vi "Ramp Down R1.vi"(10 "V":dbl, 11 "Refnum in":refnum<k20>) -> (3 "Refnum out":refnum<k20>)   [LabVIEW 2018]
uses:
  <vilib>/Utility/error.llb/Error Cluster From Error Code.vi
  <vilib>/rvi/errors/niLvFpgaAdjustHostInterfaceError.vi
  <vilib>/rvi/interface/nirviReadWriteControl/nirviReadWriteControl.xnode
  NiFpgaLv.dll
  <vilib>/rvi/interface/Simulation/niFpgaSimulationCallBeginRW.vi
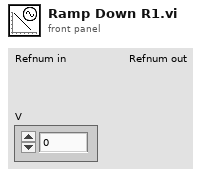
[diagram p1: front panel]
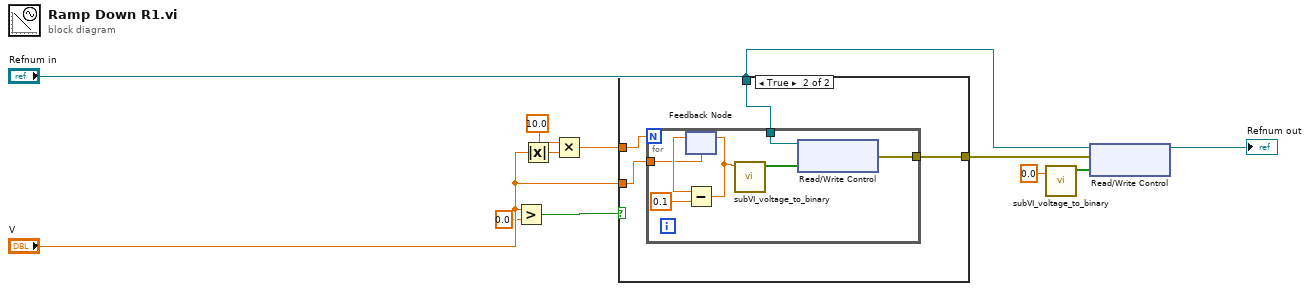
[diagram p0: block diagram]
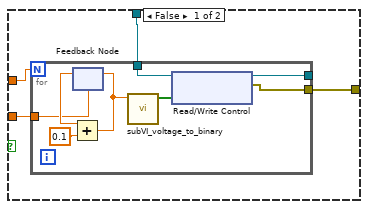
[diagram p2: hidden frame]
diagram:
  n1 = Greater?(x="V", y=0.0) -> (0:w1:bool)
  n2 = Absolute Value(x="V") -> (abs(x)=w5:dbl)
  n3 = Multiply(x=10.0, y=w5) -> (x*y=w2:dbl)
  n4 = case shown="True" w1 {
    tunnel: w2 -> [w15 w27]
    tunnel: "Refnum in" -> [w14 w26]
    tunnel: [w13 w25] -> w9
    tunnel: "V" -> [w12 w24]
    frame False {
      n5 = for {
        N: w15 -> [_]
        tunnel: [w22] -> _
        tunnel: [w18] -> w13
        tunnel: w14 -> [w17]
        tunnel: w12 -> [w16]
        n6 = feedback #1(w16) -> (w20:dbl)
        n7 = Add(x=w20, y=0.1) -> (x+y=w19:dbl)
        n8 = feedback-in #1(w19) -> ()
        n9 = call "subVI_voltage_to_binary.vi"("voltage"=w19) -> ("binary"=w23:bool[])  [unwired: 10 in]
        n10 = xnode "Read/Write Control"("FPGA VI Reference In"=w17, "DAC 1 write"=w23) -> ("FPGA VI Reference Out"=w22:refnum<k20>, "error out"=w18:errorcluster)  [unwired: 1 in]
      }
    }
    frame True {
      n11 = for {
        N: w27 -> [_]
        tunnel: [w30] -> w25
        tunnel: w26 -> [w29]
        tunnel: w24 -> [w28]
        n12 = feedback #2(w28) -> (w33:dbl)
        n13 = Subtract(x=w33, y=0.1) -> (x-y=w31:dbl)
        n14 = feedback-in #2(w31) -> ()
        n15 = call "subVI_voltage_to_binary.vi"("voltage"=w31) -> ("binary"=w34:bool[])  [unwired: 10 in]
        n16 = xnode "Read/Write Control"("FPGA VI Reference In"=w29, "DAC 2 write"=w34) -> ("error out"=w30:errorcluster)  [unwired: 1 in, 1 out]
      }
    }
  }
  n17 = call "subVI_voltage_to_binary.vi"("voltage"=0.0) -> ("binary"=w7:bool[])  [unwired: 10 in]
  n18 = xnode "Read/Write Control"("FPGA VI Reference In"="Refnum in", "error in"=w9, "DAC 1 write"=w7) -> ("FPGA VI Reference Out"=→"Refnum out":refnum<k20>)  [unwired: 1 out]
